vi "Get Address Map Element.vi"(2 "niUSRP Tx DSP v2 FPGA":refnum<class "niUSRP Tx DSP v2 FPGA.lvclass">, 5 "index":u8) -> (6 "address map element":T1)   [LabVIEW 2025, in "niUSRP Tx DSP v2 FPGA.lvclass"]
uses:
  niUSRP Tx DSP v2 FPGA.lvclass
  <instrlib>/_niInstr/Instruction Framework/v1/FPGA/Typedefs/Address Map Element.ctl
  <instrlib>/_niInstr/Instruction Framework/v1/FPGA/Typedefs/niInstr Instruction Framework v1 FPGA.lvlib
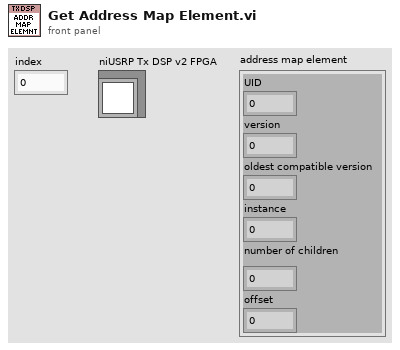
[diagram p1: front panel]
types:
  T1 = typedef "niInstr Instruction Framework v1 FPGA.lvlib/Address Map Element.ctl" = cluster{"UID":u16, "version":u16, "oldest compatible version":u16, "instance":u8, "number of children":u8, "offset":u32}
  T2 = typedef "niInstr Address Space Collection Builder v1 FPGA.lvlib/Parent Metadata.ctl" = cluster{"UID":u16, "version":u16, "oldest compatible version":u16}
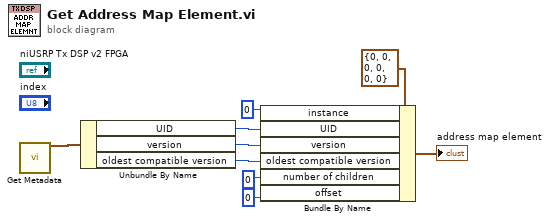
[diagram p0: block diagram]
diagram:
  n1 = call "Get Metadata.vi"() -> ("gen metadata"=w1:T2)  [unwired: 15 in]
  n2 = Unbundle By Name(w1) -> ("UID"=w7:u16, "version"=w6:u16, "oldest compatible version"=w5:u16)
  n3 = Bundle By Name(cluster=T1 {"UID"=0, "version"=0, "oldest compatible version"=0, "instance"=0, "number of children"=0, "offset"=0} ("address map element"), "instance"=u8 0, "UID"=w7, "version"=w6, "oldest compatible version"=w5, "number of children"=u8 0 ("instance"), "offset"=u32 0) -> (→"address map element":T1)
